vi "Write T Controller Settings.vi"(4 "New PID":cluster{"P":dbl, "I":dbl, "D":dbl}, 6 "Heater level":dbl, 7 "Set point":dbl, 8 "error in (no error)":errorcluster, 9 "New Heater mode":T1(ring), 10 "Hater range":dbl, 11 "Temperature controller in":refnum<class "Temperature controller.lvclass">) -> (0 "error out":errorcluster, 3 "Temperature controller out":refnum<class "Temperature controller.lvclass">)   [LabVIEW 2015, in "Temperature controller.lvclass"]
uses:
  Temperature controller.lvclass
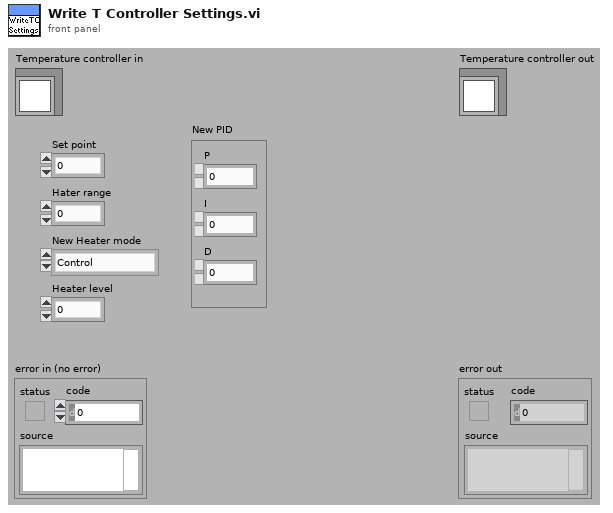
[diagram p1: front panel]
types:
  T1 = enum16{"Control", "Monitor", "Manual Heat", "Controller is in OFF mode", "Autotune is in progress"}
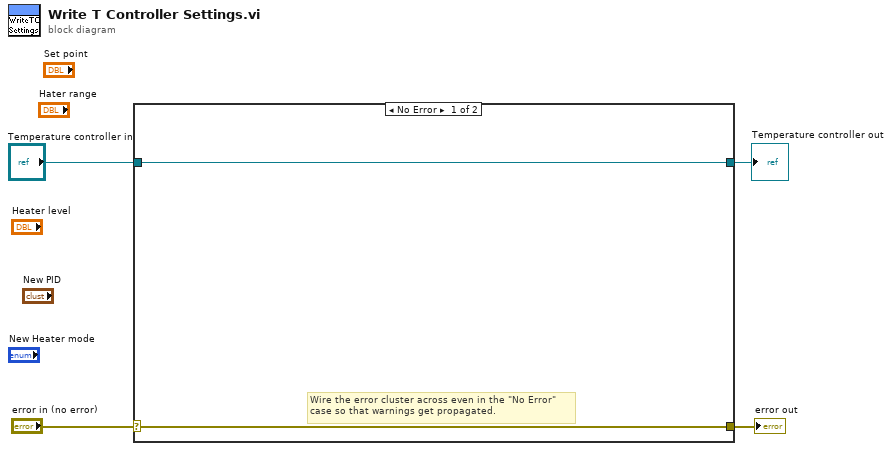
[diagram p0: block diagram]
diagram:
  n1 = case shown="No Error" "error in (no error)" {
    selector: "error in (no error)" -> [w5 w8]
    tunnel: [w5 w8] -> w3
    tunnel: [w6 w7] -> w1
    tunnel: "Temperature controller in" -> [w6 w7]
    frame No Error {
      # "Wire the error cluster across even in the \"No Error\"\ncase so that warnings get propagated."
    }
    frame Error {
    }
  }
  "error out" <- w3
  "Temperature controller out" <- w1
